vi "dfd_Mutate Filter Obj QSetting 0x100 to 0x200.vi"(11 "filter in":T1={"mSRate_Fs"=1.0, "mSRate_Version"="2.0", "mSRate_Comments"="", "mSRate_OrgCoef"={"type"=enum."Undefined", "gain"=1.0, "coef a (k)"=[], "coef b (v)"=[]}, "mSRate_CurCoef"={"type"=enum."Undefined", "gain"=1.0, "coef a (k)"=[], "coef b (v)"=[]}, "mSRate_Quantized?"=FALSE, "mSRate_QCoef"={"type"=enum."Undefined", "gain"=1.0, "coef a (k)"=[], "coef b (v)"=[]}, "mSRate_QSettings"=[], "mSRate_Order"=0, "mSRate_Scaling"={"mSRate_ScaleByPowerOf2?"=FALSE, "mSRate_ScaleType"=enum."No Norm"}} {"mSRate_QSettings"."source" items=["Coef a/k"=0, "Coef b/v"=7, "Input"=1, "Output"=2, "Multiplicand"=3, "Product"=4, "Sum"=5, "Delay"=6, "Gain"=8]}) -> (3 "filter out":T1={"mSRate_Fs"=1.0, "mSRate_Version"="2.0", "mSRate_Comments"="", "mSRate_OrgCoef"={"type"=enum."Undefined", "gain"=1.0, "coef a (k)"=[], "coef b (v)"=[]}, "mSRate_CurCoef"={"type"=enum."Undefined", "gain"=1.0, "coef a (k)"=[], "coef b (v)"=[]}, "mSRate_Quantized?"=FALSE, "mSRate_QCoef"={"type"=enum."Undefined", "gain"=1.0, "coef a (k)"=[], "coef b (v)"=[]}, "mSRate_QSettings"=[], "mSRate_Order"=0, "mSRate_Scaling"={"mSRate_ScaleByPowerOf2?"=FALSE, "mSRate_ScaleType"=enum."No Norm"}} {"mSRate_QSettings"."source" items=["Coef a/k"=0, "Coef b/v"=7, "Input"=1, "Output"=2, "Multiplicand"=3, "Product"=4, "Sum"=5, "Delay"=6, "Gain"=8]})   [LabVIEW 2017]
uses:
  <vilib>/addons/Digital Filter Design/_Objects.llb/DFD Filter Obj.ctl
  <vilib>/addons/Digital Filter Design/_Objects.llb/DFD Filter Coef.ctl
  <vilib>/addons/Digital Filter Design/_Objects.llb/DFD Filter Structure Type Selector.ctl
  <vilib>/addons/Digital Filter Design/_Objects.llb/dfd_Internal Quantization Settings.ctl
  <vilib>/addons/Digital Filter Design/_Objects.llb/dfd_Internal Quantization Srcs.ctl
  <vilib>/addons/Digital Filter Design/_Objects.llb/DFD Coef Norm Type.ctl
  <vilib>/addons/Digital Filter Design/FilterLib.llb/dfd_Get Filter Coef Type (Filter IO).vi
  <vilib>/addons/Digital Filter Design/NI_DigFilterLicensed.lvlib
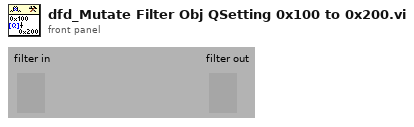
[diagram p1: front panel]
types:
  T1 = typedef "NI_DigFilterLicensed.lvlib/DFD Filter Obj.ctl" = cluster{"mSRate_Fs":dbl, "mSRate_Version":string, "mSRate_Comments":string, "mSRate_OrgCoef":T2, "mSRate_CurCoef":T2, "mSRate_Quantized?":bool, "mSRate_QCoef":T2, "mSRate_QSettings":T4[], "mSRate_Order":i32, "mSRate_Scaling":cluster{"mSRate_ScaleByPowerOf2?":bool, "mSRate_ScaleType":T6}}
  T2 = typedef "NI_DigFilterLicensed.lvlib/DFD Filter Coef.ctl" = cluster{"type":T3, "gain":dbl, "coef a (k)":dbl[], "coef b (v)":dbl[]}
  T3 = typedef "NI_DigFilterLicensed.lvlib/DFD Filter Structure Type Selector.ctl" = enum16{"Undefined", "FIR Direct Form", "FIR Direct Form Transposed", "FIR Symmetric", "FIR Antisymmetric", "IIR Direct Form I", "IIR Direct Form I Transposed", "IIR Direct Form II", "IIR Direct Form II Transposed", "IIR Cascaded Second Order Sections Form I", "IIR Cascaded Second Order Sections Form I Transposed", "IIR Cascaded Second Order Sections Form II", "IIR Cascaded Second Order Sections Form II Transposed", "Lattice Allpass (basic sections)", "Lattice Allpass (one multiplier sections)", "Lattice Allpass (normalized sections)", "Lattice AR (basic sections)", "Lattice AR (one multiplier sections)", "Lattice AR (normalized sections)", "Lattice MA (minimum phase)", "Lattice MA (maximum phase)", "Lattice ARMA (basic sections)", "Lattice ARMA (one multiplier sections)", "Lattice ARMA (normalized sections)"}
  T4 = typedef "NI_DigFilterLicensed.lvlib/dfd_Internal Quantization Settings.ctl" = cluster{"source":T5, "wl":i16, "iwl":i16, "overflow mode":enum16{"Saturation", "Wrap"}, "rounding mode":enum16{"Nearest", "Truncation"}, "signed?":bool}
  T5 = typedef "NI_DigFilterLicensed.lvlib/dfd_Internal Quantization Srcs.ctl" = u16
  T6 = typedef "NI_DigFilterLicensed.lvlib/DFD Coef Norm Type.ctl" = enum16{"No Norm", "Time Domain 1-Norm", "Time Domain 2-Norm", "Time Domain Inf-Norm"}
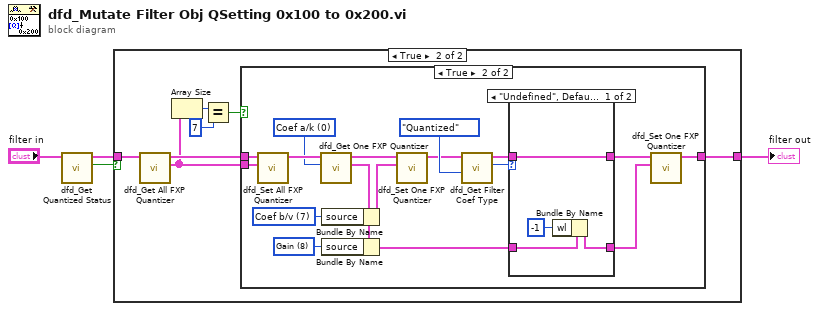
[diagram p0: block diagram]
diagram:
  n1 = call <vilib>:"dfd_Get Quantized Status.vi"("filter in"="filter in") -> ("quantized?"=w2:bool, "filter out"=w3:T1)  [unwired: 1 in, 8 out]
  n2 = case shown="True" w2 {
    tunnel: w3 -> [w5 w12]
    tunnel: [w5 w10] -> w1
    frame False {
    }
    frame True {
      n3 = call <vilib>:"dfd_Get All FXP Quantizer.vi"("filter in"=w12) -> ("quantization settings"=w9:T4[], "filter out"=w11:T1)  [unwired: 1 in, 8 out]
      n4 = Array Size(array=w9) -> (size(s)=w8:i32)
      n5 = Equal?(x=w8, y=7) -> (x = y?=w6:bool)
      n6 = case shown="True" w6 {
        tunnel: w11 -> [w13 w30]
        tunnel: [w13 w16] -> w10
        tunnel: w9 -> [_ w14]
        frame False {
        }
        frame True {
          w26 = T5 8 items=["Coef a/k"=0, "Coef b/v"=7, "Input"=1, "Output"=2, "Multiplicand"=3, "Product"=4, "Sum"=5, "Delay"=6, "Gain"=8] ("source")
          w27 = T5 7 items=["Coef a/k"=0, "Coef b/v"=7, "Input"=1, "Output"=2, "Multiplicand"=3, "Product"=4, "Sum"=5, "Delay"=6, "Gain"=8] ("source")
          w28 = T5 0 items=["Coef a/k"=0, "Coef b/v"=7, "Input"=1, "Output"=2, "Multiplicand"=3, "Product"=4, "Sum"=5, "Delay"=6, "Gain"=8] ("quantization source")
          n7 = call <vilib>:"dfd_Set All FXP Quantizer.vi"("quantization settings"=w14, "filter in"=w30) -> ("filter out"=w29:T1)  [unwired: 1 in, 8 out]
          n8 = call <vilib>:"dfd_Get One FXP Quantizer.vi"("quantization source"=w28, "filter in"=w29) -> ("quantization settings"=w20:T4, "filter out"=w25:T1)  [unwired: 1 in, 7 out]
          n9 = Bundle By Name(cluster=w20, "source"=w27) -> (w19:T4)
          n10 = Bundle By Name(cluster=w20, "source"=w26) -> (w18:T4)
          n11 = call <vilib>:"dfd_Set One FXP Quantizer.vi"("quantization settings"=w19, "filter in"=w25) -> ("filter out"=w23:T1)  [unwired: 1 in, 8 out]
          n12 = call-poly <vilib>:"dfd_Get Filter Coef Type.vi"("coef source"=enum16{"Original", "Current", "Quantized"}."Quantized", "filter in"=w23) -> ("type"=w22:T3, "filter out"=w21:T1)  [unwired: 2 in, 6 out]
          n13 = case shown="\"Undefined\", Default" w22 {
            tunnel: w21 -> [w32 w36]
            tunnel: w18 -> [w34 w35]
            tunnel: [w32 w36] -> w17
            tunnel: [w31 w35] -> w15
            frame "Undefined", Default {
              n14 = Bundle By Name(cluster=w34, "wl"=i16 -1) -> (w31:T4)
            }
            frame "Lattice AR (basic sections)".."Lattice MA (maximum phase)" {
            }
          }
          n15 = call <vilib>:"dfd_Set One FXP Quantizer.vi"("quantization settings"=w15, "filter in"=w17) -> ("filter out"=w16:T1)  [unwired: 1 in, 8 out]
        }
      }
    }
  }
  "filter out" <- w1
